vi "autoqueue_dynamic_DUAL.vi"(0 "cluster":T5, 1 "1to4":T3, 4 "xy dynamic array":T1(array[cluster]), 5 "error out":errorcluster, 6 "output cluster":T4, 7 "reference":refnum<vi>, 9 "index":dbl format="%#_13g", 10 "last tme":dbl format="%#_13g", 11 "Str Refnum":refnum<vi>, 12 "Cluster":cluster{"1":bool, "2":bool}, 13 "reference 2":refnum<vi>, 14 "Report Data.Degree":dbl[][](array[numeric])) -> (19 "error out 2":errorcluster)   [LabVIEW 2015]
uses:
  Typedef/Inst. Queue.ctl
  Typedef/State.ctl
panel:
  in  "Array  1":T2(array[cluster])
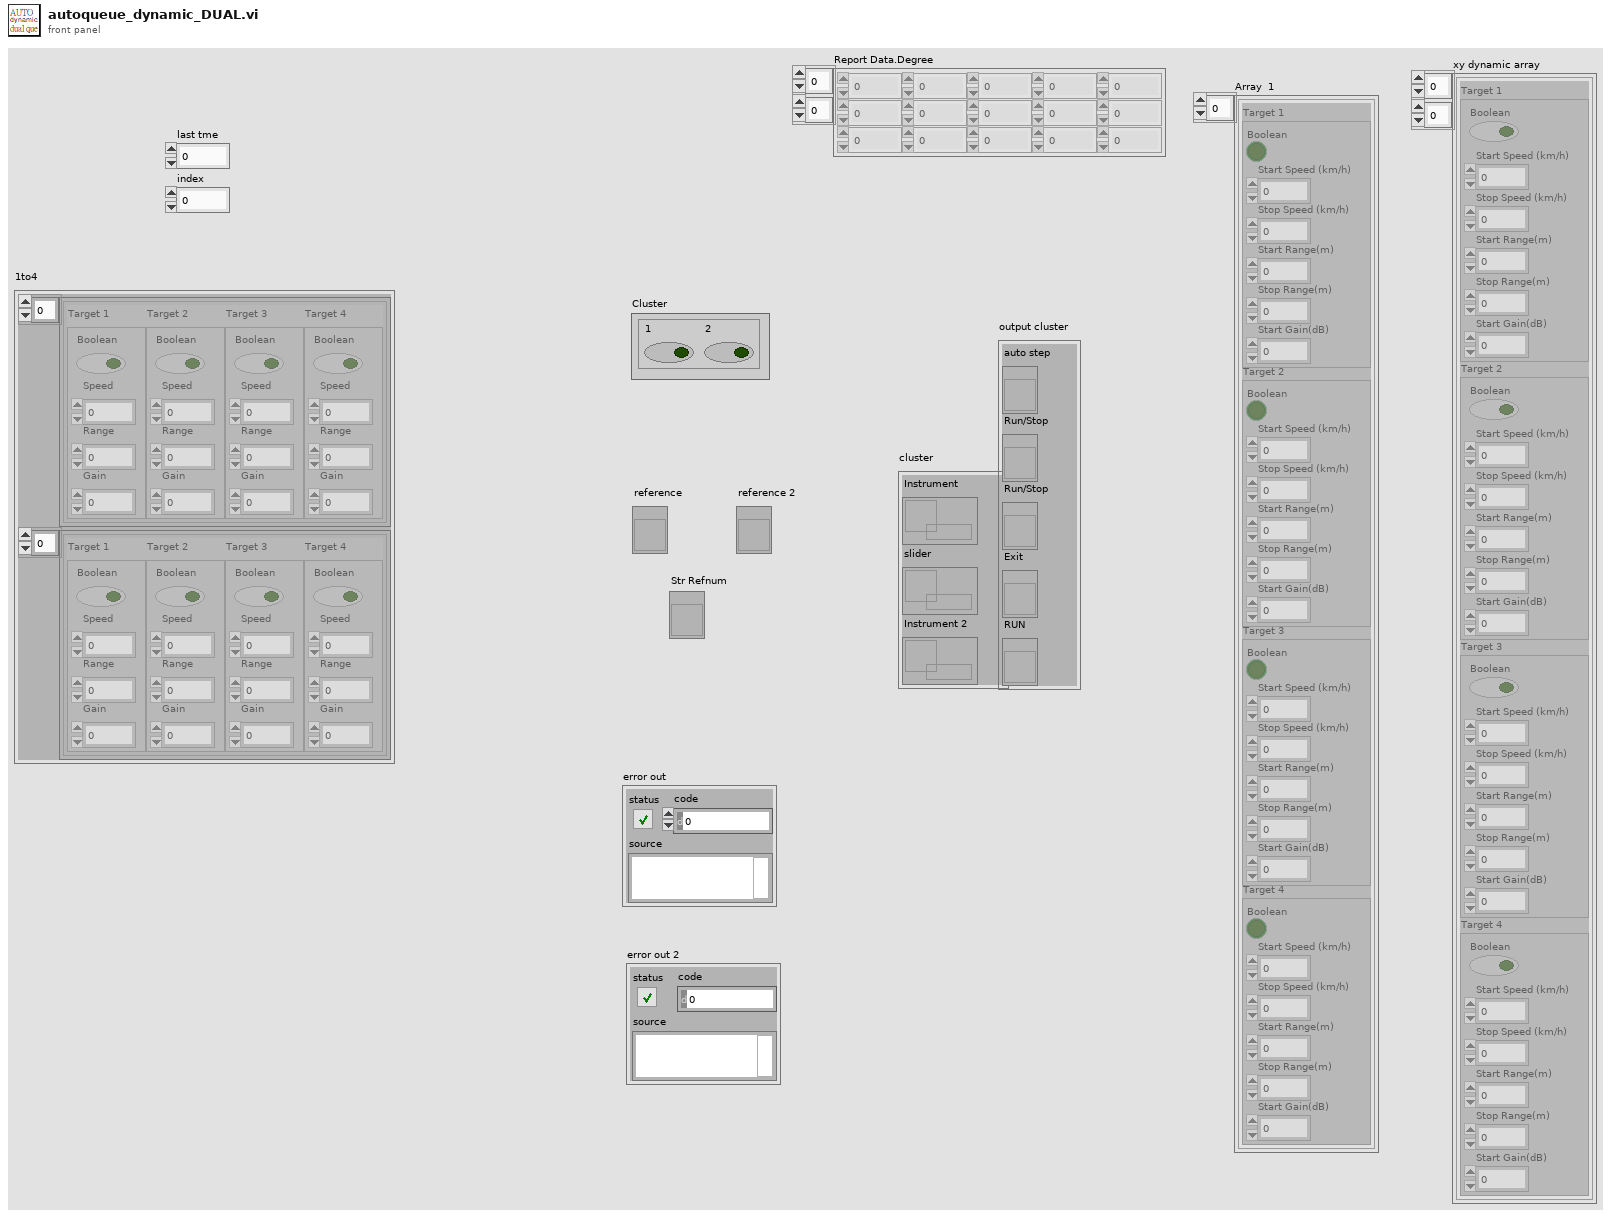
[diagram p1: front panel]
types:
  T1 = cluster{"Target 1":cluster{"Boolean":bool, "Start Speed (km/h)":dbl, "Stop Speed (km/h)":dbl, "Start Range(m)":dbl, "Stop Range(m)":dbl, "Start Gain(dB)":dbl}, "Target 2":cluster{"Boolean":bool, "Start Speed (km/h)":dbl, "Stop Speed (km/h)":dbl, "Start Range(m)":dbl, "Stop Range(m)":dbl, "Start Gain(dB)":dbl}, "Target 3":cluster{"Boolean":bool, "Start Speed (km/h)":dbl, "Stop Speed (km/h)":dbl, "Start Range(m)":dbl, "Stop Range(m)":dbl, "Start Gain(dB)":dbl}, "Target 4":cluster{"Boolean":bool, "Start Speed (km/h)":dbl, "Stop Speed (km/h)":dbl, "Start Range(m)":dbl, "Stop Range(m)":dbl, "Start Gain(dB)":dbl}}[][]
  T2 = cluster{"Target 1":cluster{"Boolean":bool, "Start Speed (km/h)":dbl, "Stop Speed (km/h)":dbl, "Start Range(m)":dbl, "Stop Range(m)":dbl, "Start Gain(dB)":dbl}, "Target 2":cluster{"Boolean":bool, "Start Speed (km/h)":dbl, "Stop Speed (km/h)":dbl, "Start Range(m)":dbl, "Stop Range(m)":dbl, "Start Gain(dB)":dbl}, "Target 3":cluster{"Boolean":bool, "Start Speed (km/h)":dbl, "Stop Speed (km/h)":dbl, "Start Range(m)":dbl, "Stop Range(m)":dbl, "Start Gain(dB)":dbl}, "Target 4":cluster{"Boolean":bool, "Start Speed (km/h)":dbl, "Stop Speed (km/h)":dbl, "Start Range(m)":dbl, "Stop Range(m)":dbl, "Start Gain(dB)":dbl}}[]
  T3 = cluster{cluster{"Target 1":cluster{"Boolean":bool, "Speed":dbl, "Range":dbl, "Gain":dbl}, "Target 2":cluster{"Boolean":bool, "Speed":dbl, "Range":dbl, "Gain":dbl}, "Target 3":cluster{"Boolean":bool, "Speed":dbl, "Range":dbl, "Gain":dbl}, "Target 4":cluster{"Boolean":bool, "Speed":dbl, "Range":dbl, "Gain":dbl}}[], cluster{"Target 1":cluster{"Boolean":bool, "Speed":dbl, "Range":dbl, "Gain":dbl}, "Target 2":cluster{"Boolean":bool, "Speed":dbl, "Range":dbl, "Gain":dbl}, "Target 3":cluster{"Boolean":bool, "Speed":dbl, "Range":dbl, "Gain":dbl}, "Target 4":cluster{"Boolean":bool, "Speed":dbl, "Range":dbl, "Gain":dbl}}[]}
  T4 = cluster{"auto step":refnum<vi>, "Run/Stop":refnum<vi>, "Run/Stop":refnum<vi>, "Exit":refnum<vi>, "RUN":refnum<vi>}
  T5 = cluster{"Instrument":refnum<queue>, "slider":refnum<queue>, "Instrument 2":refnum<queue>}
  T6 = typedef "Inst. Queue.ctl" = cluster{enum16{"auto mode", "Idle", "Inst. Connect", "£m Data", "Inst. Update", "Freq. (GHz)", "rx att", "GTX (dB)", "GRX (dB)", "Range Trim(m)", "Gain Trim (dB)", "Distance to RUT", "Mapping", "Convert", "RF ON/OFF", "Run", "Direct Program", "Stop", "Dynamic", "dyset", "Exit"}, "variant":variant}
  T7 = typedef "State.ctl" = enum16{"Idle", "Initial", "Update", "get angle", "Axis", "Connect", "Creep", "Speed", "Distance", "Move Method", "Move Mode", "Direct of Movement", "Initail Speed", "Sramp", "Normal Open", "Acceleration", "Deceleration", "Angle", "Move&Rotate", "Rotate", "Rotate_2", "Return to Origin", "Move", "Inching", "Return to Zero", "Return to Middle", "Go to Step1", "Go to Step2", "Go to Step3", "Initial to Y Step", "Select Speed", "auto mode", "Stop", "reset xy", "reset ant", "set speed", "Exit"}
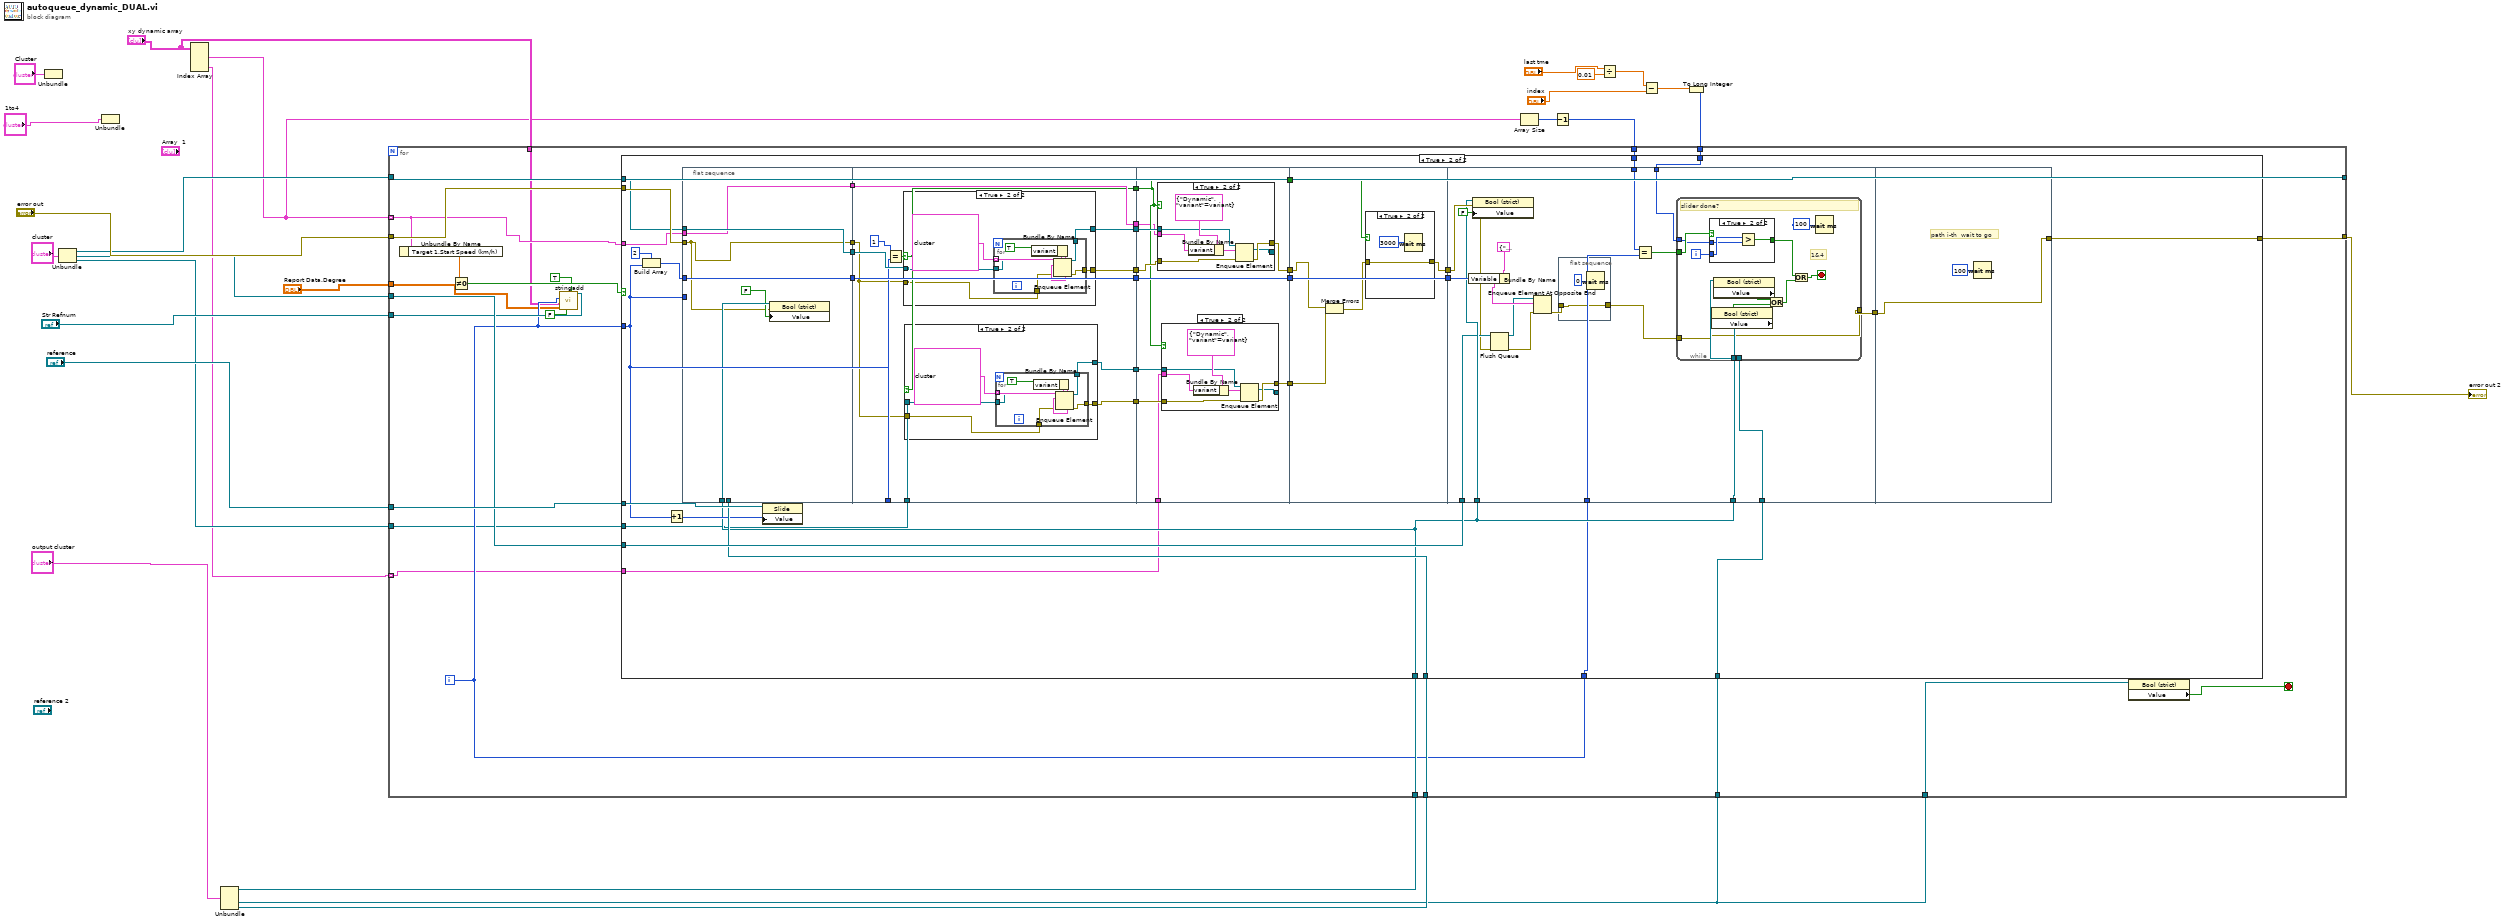
[diagram p0: block diagram]
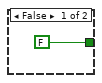
[diagram p8: hidden frame]
diagram:
  n1 = Unbundle("Cluster") -> ()  [unwired: 2 out]
  n2 = Unbundle("cluster") -> ("Instrument"=w24:refnum<queue>, "slider"=w23:refnum<queue>, "Instrument 2"=w13:refnum<queue>)
  n3 = Unbundle("1to4") -> ()  [unwired: 2 out]
  n4 = Index Array(array="xy dynamic array") -> (element #1=w9:T2, element #2=w10:T2)  [unwired: 4 in]
  n5 = Unbundle("output cluster") -> ("auto step"=w17:refnum<vi>, "Exit"=w16:refnum<vi>, "RUN"=w18:refnum<vi>)  [unwired: 2 out]
  n6 = Array Size(array=w9) -> (size(s)=w2:i32)
  n7 = Decrement(x=w2) -> (x-1=w1:i32)
  n8 = Divide(x="last tme", y=0.01) -> (x/y=w7:dbl)
  n9 = Subtract(x=w7, y="index") -> (x-y=w6:dbl)
  n10 = To Long Integer(number=w6) -> (32bit integer=w3:i32)
  n11 = for {
    tunnel: w24 -> [w46]
    tunnel: w23 -> [w45]
    tunnel: "reference" -> [w47]
    tunnel: [w46] -> _
    tunnel: w18 -> [w40]
    tunnel: w17 -> [w41]
    tunnel: w16 -> [w44]
    tunnel: w16 -> [w43]
    tunnel: "Str Refnum" -> [w36]
    tunnel: "error out" -> [w48]
    tunnel: [w49] -> w11
    tunnel: "Report Data.Degree" -> [w31]
    tunnel: w9 -> [w33] mode=indexing
    tunnel: w13 -> [w32]
    tunnel: w10 -> [w30] mode=indexing
    tunnel: "xy dynamic array" -> [w29]
    tunnel: w1 -> [w28]
    tunnel: w3 -> [w27]
    i -> [w34]
    stop <- w42 stop-if-true
    n12 = Unbundle By Name(w33) -> ("Target 1.Start Speed (km/h)"=w39:dbl)
    n13 = Not Equal To 0?(x=w39) -> (x != 0?=w38:bool)
    n14 = call "stringadd.vi"("Report Data.Degree"=w31, "Mode"=TRUE, "s/d setting"=FALSE, "Str Refnum"=w36, "variant"=w29, "Numeric"=w34) -> ()  [unwired: 6 in]
    n15 = case shown="True" w38 {
      tunnel: [w50 w74] -> w49
      tunnel: w48 -> [w50 w86]
      tunnel: w47 -> [_ w85]
      tunnel: w46 -> [_ w84]
      tunnel: w45 -> [_ w83]
      tunnel: w44 -> [_ w78]
      tunnel: w34 -> [_ w72]
      tunnel: w41 -> [_ w59]
      tunnel: w40 -> [_ w82]
      tunnel: w33 -> [_ w81]
      tunnel: w34 -> [_ w53]
      tunnel: w32 -> [_ w58]
      tunnel: w30 -> [_ w54]
      tunnel: w28 -> [_ w52]
      tunnel: w27 -> [_ w51]
      frame False {
      }
      frame True {
        n16 = Build Array(2 ("element"), w72) -> (w73:i32[])
        n17 = Increment(x=w72) -> (x+1=w80:i32)
        n18 = flat-sequence {
          tunnel: w73 -> [w92]
          tunnel: w86 -> [w87]
          tunnel: w84 -> [w89]
          tunnel: w81 -> [w88]
          tunnel: [w92] -> w77
          tunnel: w59 -> [w91]
          tunnel: w82 -> [_]
          tunnel: [w87] -> w76
          tunnel: w72 -> [_]
          tunnel: [w89] -> w67
          tunnel: [w88] -> w65
          tunnel: w77 -> [w104]
          tunnel: [w104] -> w71
          tunnel: w76 -> [w97]
          tunnel: [w103] -> w70
          tunnel: w72 -> [w101]
          tunnel: [w100] -> w69
          tunnel: [w96] -> w68
          tunnel: w67 -> [w102]
          tunnel: [w99] -> w66
          tunnel: w65 -> [w99]
          tunnel: w58 -> [w95]
          tunnel: [w94] -> w57
          tunnel: [w93] -> w56
          tunnel: w71 -> [w142]
          tunnel: [w142] -> w64
          tunnel: w70 -> [w140]
          tunnel: [w139] -> w62
          tunnel: w69 -> [w141]
          tunnel: w68 -> [w138]
          tunnel: w66 -> [w136]
          tunnel: [w138] -> w60
          tunnel: w57 -> [w137]
          tunnel: w56 -> [w135]
          tunnel: [w134] -> w55
          tunnel: w54 -> [w133]
          tunnel: w64 -> [w166]
          tunnel: [w166] -> w63
          tunnel: w62 -> [w163]
          tunnel: [w165] -> w61
          tunnel: w60 -> [w164]
          tunnel: w55 -> [w162]
          tunnel: w83 -> [w176]
          tunnel: w63 -> [w187]
          tunnel: w59 -> [w185]
          tunnel: w78 -> [w184]
          tunnel: [w183] -> w75
          tunnel: w61 -> [w180]
          tunnel: w59 -> [w179]
          tunnel: w53 -> [w172]
          tunnel: w52 -> [w173]
          tunnel: w51 -> [w171]
          tunnel: w75 -> [w208]
          tunnel: [w208] -> w74
          frame #0 {
            n19 = property on="Property Node" class="Bool (strict)"(reference=w91, error in=w87, "Value"=FALSE) -> ()  [unwired: 2 out]
          }
          frame #1 {
            n20 = Equal?(x=1 ("element"), y=w101) -> (x = y?=w96:bool)
            n21 = case shown="True" w96 {
              tunnel: [w120 w125] -> w103
              tunnel: w97 -> [w120 w124]
              tunnel: w102 -> [w119 w123]
              tunnel: [w119 w121] -> w100
              frame False {
              }
              frame True {
                n22 = for {
                  tunnel: T6[] [{enum."Convert", "variant"=variant}, {enum."RF ON/OFF", "variant"=variant}] -> [w131] mode=indexing
                  tunnel: [w132] -> w125
                  tunnel: w124 -> [w128]
                  tunnel: w123 -> [w127]
                  tunnel: [w126] -> w121
                  n23 = Bundle By Name(cluster=w131, "variant"=TRUE) -> (w130:T6)
                  n24 = Enqueue Element(queue=w127, element=w130, error in (no error)=w128) -> (queue out=w126:refnum<queue>, error out=w132:errorcluster)  [unwired: 1 in, 1 out]
                }
              }
            }
            n25 = case shown="True" w96 {
              tunnel: [w106 w111] -> w93
              tunnel: w97 -> [w106 w110]
              tunnel: w95 -> [w105 w109]
              tunnel: [w105 w107] -> w94
              frame False {
              }
              frame True {
                n26 = for {
                  tunnel: T6[] [{enum."Convert", "variant"=variant}, {enum."RF ON/OFF", "variant"=variant}] -> [w117] mode=indexing
                  tunnel: [w118] -> w111
                  tunnel: w110 -> [w114]
                  tunnel: w109 -> [w113]
                  tunnel: [w112] -> w107
                  n27 = Bundle By Name(cluster=w117, "variant"=TRUE) -> (w116:T6)
                  n28 = Enqueue Element(queue=w113, element=w116, error in (no error)=w114) -> (queue out=w112:refnum<queue>, error out=w118:errorcluster)  [unwired: 1 in, 1 out]
                }
              }
            }
          }
          frame #2 {
            n29 = case shown="True" w138 {
              tunnel: [w153 w159] -> w139
              tunnel: w136 -> [_ w158]
              tunnel: w141 -> [w152 w156]
              tunnel: [w152 w155] -> _
              tunnel: w140 -> [w153 w154]
              frame False {
              }
              frame True {
                n30 = Bundle By Name(cluster=T6 {enum."Dynamic", "variant"=variant}, "variant"=w158) -> (w160:T6)
                n31 = Enqueue Element(queue=w156, element=w160, error in (no error)=w154) -> (queue out=w155:refnum<queue>, error out=w159:errorcluster)  [unwired: 1 in, 1 out]
              }
            }
            n32 = case shown="True" w138 {
              tunnel: [w144 w150] -> w134
              tunnel: w133 -> [_ w149]
              tunnel: w137 -> [w143 w147]
              tunnel: [w143 w146] -> _
              tunnel: w135 -> [w144 w145]
              frame False {
              }
              frame True {
                n33 = Bundle By Name(cluster=T6 {enum."Dynamic", "variant"=variant}, "variant"=w149) -> (w151:T6)
                n34 = Enqueue Element(queue=w147, element=w151, error in (no error)=w145) -> (queue out=w146:refnum<queue>, error out=w150:errorcluster)  [unwired: 1 in, 1 out]
              }
            }
          }
          frame #3 {
            n35 = Merge Errors(w163, w162) -> (w161:errorcluster)
            n36 = case shown="True" w164 {
              tunnel: w161 -> [w167 w169]
              tunnel: [w167 w169] -> w165
              frame False {
              }
              frame True {
                n37 = Wait (ms)(milliseconds to wait=u32 3000) -> ()  [unwired: 1 out]
              }
            }
          }
          frame #4 {
            n38 = Bundle By Name(cluster=cluster{"State":T7, "Variable":variant} {"State"=enum."auto mode", "Variable"=variant}, "Variable"=w187) -> (w186:cluster{"State":T7, "Variable":variant})
            n39 = property class="Bool (strict)"(reference=w179, error in=w180, "Value"=FALSE) -> (error out=w174:errorcluster)  [unwired: 1 out]
            n40 = Flush Queue(queue=w176, error in (no error)=w174) -> (queue out=w175:refnum<queue>, error out=w177:errorcluster)  [unwired: 1 out]
            n41 = Enqueue Element At Opposite End(queue=w175, element=w186, error in (no error)=w177) -> (error out=w182:errorcluster)  [unwired: 1 in, 2 out]
            n42 = flat-sequence {
              tunnel: w182 -> [w190]
              tunnel: [w190] -> w181
              frame #0 {
                n43 = Wait (ms)(milliseconds to wait=u32 0) -> ()  [unwired: 1 out]
              }
            }
            n44 = Equal?(x=w173, y=w172) -> (x = y?=w170:bool)
            n45 = while {
              tunnel: [w197] -> w183
              tunnel: w184 -> [w199]
              tunnel: w185 -> [w198]
              tunnel: w181 -> [w197]
              tunnel: w171 -> [w191]
              tunnel: w170 -> [w196]
              i -> [w192]
              stop <- w195 stop-if-true
              # "1&4"
              # "slider done?"
              n46 = case shown="True" w196 {
                tunnel: [FALSE w204] -> w193
                tunnel: w192 -> [_ w206]
                tunnel: w191 -> [_ w205]
                frame False {
                }
                frame True {
                  n47 = Greater?(x=w206, y=w205) -> (0:w204:bool)
                }
              }
              n48 = property on="Property Node" class="Bool (strict)"(reference=w198) -> ("Value"=w200:bool)  [unwired: 1 in, 2 out]
              n49 = property on="Property Node" class="Bool (strict)"(reference=w199) -> ("Value"=w201:bool)  [unwired: 1 in, 2 out]
              n50 = Or(x=w201, y=w200) -> (x .or. y?=w194:bool)
              n51 = Or(x=w193, y=w194) -> (x .or. y?=w195:bool)
              n52 = Wait (ms)(milliseconds to wait=u32 100) -> ()  [unwired: 1 out]
            }
          }
          frame #5 {
            # "path i-th  wait to go"
            n53 = Wait (ms)(milliseconds to wait=u32 100) -> ()  [unwired: 1 out]
          }
        }
        n54 = property class="Slide"(reference=w85, "Value"=w80) -> ()  [unwired: 1 in, 2 out]
      }
    }
    n55 = property on="Property Node" class="Bool (strict)"(reference=w43) -> ("Value"=w42:bool)  [unwired: 1 in, 2 out]
  }
  "error out 2" <- w11
